vi "overhaul.vi"(9 "goal node reference":refnum<data-value>, 10 "start node reference":refnum<data-value>, 11 "AD* in":refnum<class "NI_Robotics_AnytimeDStar.lvclass">) -> (3 "AD* out":refnum<class "NI_Robotics_AnytimeDStar.lvclass">)   [LabVIEW 2017, in "NI_Robotics_AnytimeDStar.lvclass"]
uses:
  <vilib>/robotics/Navigation/Anytime D Star/NI_Robotics_AnytimeDStar.lvclass
  <vilib>/robotics/Navigation/shared/MapNode/AbstractDstarNode/NI_Robotics_AbstractDstarNode.lvclass
  <vilib>/robotics/Navigation/Anytime D Star/NI_Robotics_AnytimeDStar.lvclass/NI_Robotics_AnytimeDStar.ctl
  <vilib>/robotics/Navigation/shared/Priority Queue/NI_Robotics_Priority Queue.lvclass
  <vilib>/robotics/Navigation/shared/InconsistentList/NI_Robotics_InconsistentList.lvclass
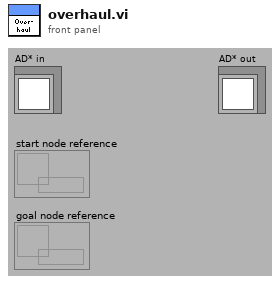
[diagram p1: front panel]
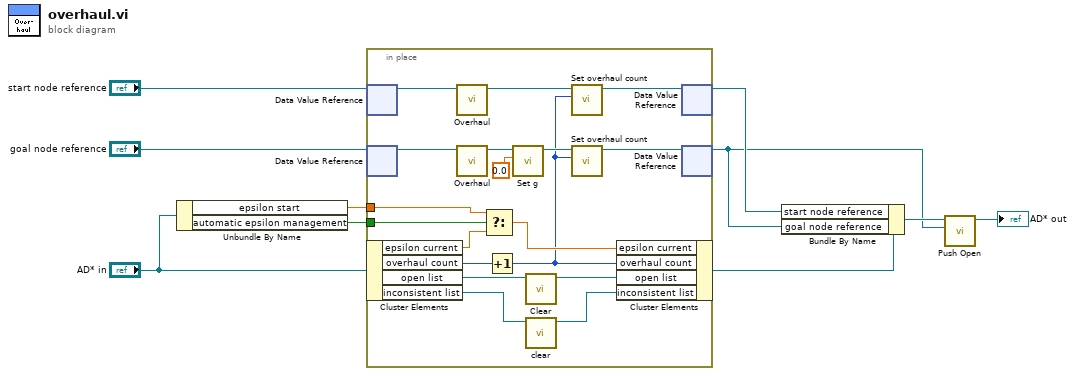
[diagram p0: block diagram]
diagram:
  n1 = Unbundle By Name("AD* in") -> ("epsilon start"=w5:dbl, "automatic epsilon management"=w6:bool)
  n2 = in-place {
    in-place-border: w6 -> [w23]
    in-place-border: w5 -> [w22]
    n3 = in-place-dvr #1("start node reference") -> (w18:refnum<class "NI_Robotics_AbstractDstarNode.lvclass">)  [unwired: 1 out]
    n4 = in-place-dvr #2("goal node reference") -> (w13:refnum<class "NI_Robotics_AbstractDstarNode.lvclass">)  [unwired: 1 out]
    n5 = in-place-cluster #3("AD* in") -> ("epsilon current"=w20:dbl, "overhaul count"=w28:i32, "open list"=w27:refnum<class "NI_Robotics_Priority Queue.lvclass">, "inconsistent list"=w25:refnum<class "NI_Robotics_InconsistentList.lvclass">)
    n6 = call <vilib>:"Overhaul.vi"("AbstractDstarNode in"=w18) -> ("AbstractDstarNode out"=w19:refnum<class "NI_Robotics_AbstractDstarNode.lvclass">)  [unwired: 10 in]
    n7 = call <vilib>:"Overhaul.vi"("AbstractDstarNode in"=w13) -> ("AbstractDstarNode out"=w15:refnum<class "NI_Robotics_AbstractDstarNode.lvclass">)  [unwired: 10 in]
    n8 = Select(t=w22, s=w23, f=w20) -> (s? t:f=w21:dbl)
    n9 = Increment(x=w28) -> (x+1=w11:i32)
    n10 = call <vilib>:"Set g.vi"("g"=0.0, "AbstractDstarNode in"=w15) -> ("AbstractDstarNode out"=w16:refnum<class "NI_Robotics_AbstractDstarNode.lvclass">)  [unwired: 9 in]
    n11 = call <vilib>:"Clear.vi"("Priority Queue in"=w27) -> ("Priority Queue out"=w26:refnum<class "NI_Robotics_Priority Queue.lvclass">)  [unwired: 8 in, 2 out]
    n12 = call <vilib>:"clear.vi"("InconsistentList in"=w25) -> ("InconsistentList out"=w24:refnum<class "NI_Robotics_InconsistentList.lvclass">)  [unwired: 9 in, 1 out]
    n13 = call <vilib>:"Set overhaul count.vi"("overhaul count"=w11, "AbstractDstarNode in"=w19) -> ("AbstractDstarNode out"=w17:refnum<class "NI_Robotics_AbstractDstarNode.lvclass">)  [unwired: 9 in]
    n14 = call <vilib>:"Set overhaul count.vi"("overhaul count"=w11, "AbstractDstarNode in"=w16) -> ("AbstractDstarNode out"=w12:refnum<class "NI_Robotics_AbstractDstarNode.lvclass">)  [unwired: 9 in]
    n15 = in-place-cluster #3("epsilon current"=w21, "overhaul count"=w11, "open list"=w26, "inconsistent list"=w24) -> (w9:refnum<class "NI_Robotics_AnytimeDStar.lvclass">)
    n16 = in-place-dvr #1(w17) -> (w3:refnum<data-value>)  [unwired: 1 out]
    n17 = in-place-dvr #2(w12) -> (w1:refnum<data-value>)  [unwired: 1 out]
  }
  n18 = Bundle By Name(cluster=w9, "start node reference"=w3, "goal node reference"=w1) -> (w8:refnum<class "NI_Robotics_AnytimeDStar.lvclass">)
  n19 = call <vilib>:"Push Open.vi"("node ref in"=w1, "AD* in"=w8) -> ("AD* out"=→"AD* out":refnum<class "NI_Robotics_AnytimeDStar.lvclass">)  [unwired: 8 in, 1 out]
